vi "GA_DisplaySolution.vi"(5 "ClassifierClass.lvclass":refnum<class "ClassifierClass.lvclass">, 8 "Stop Notifier In":refnum<notifier>, 10 "Controls Refs":T1, 11 "Solution Notifier In":refnum<notifier>) -> ()   [LabVIEW 2016, in "GA.lvlib"]
uses:
  GA.lvlib
  GA_tSolution progress.ctl
  4. Accuracy Assessment for EEG Classification/_vlib/ClassifierClass.lvclass
  4. Accuracy Assessment for EEG Classification/_vlib/CU_DataTypes.ctl
  4. Accuracy Assessment for EEG Classification/Classifier.lvlib
panel:
  # "This VI is a part of BCI Design library, http://www.ru-bci.org \nCopyright © 2020, Sotnikov Peter, All rights reserved. License: GNU GPLv3"
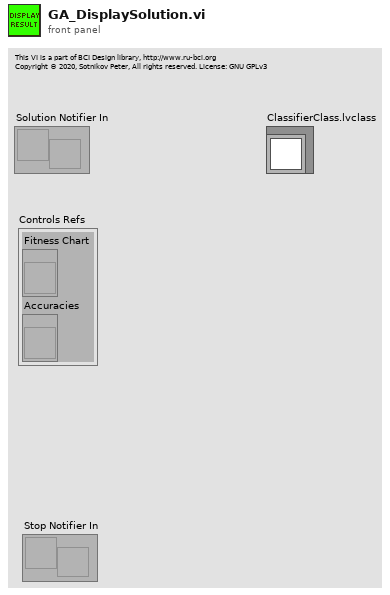
[diagram p1: front panel]
types:
  T1 = cluster{"Fitness Chart":refnum<vi>, "Accuracies":refnum<vi>}
  T2 = typedef "Classifier.lvlib/CU_DataTypes.ctl" = enum16{"Training Data", "Test Data", "Training Data (cross-check)", "Test Data (cross-check)"}
  T3 = typedef "GA.lvlib/GA_tSolution progress.ctl" = cluster{"Solution":i8[], "Fitness":dbl, "Mutation rate":dbl, "Generation":i32}
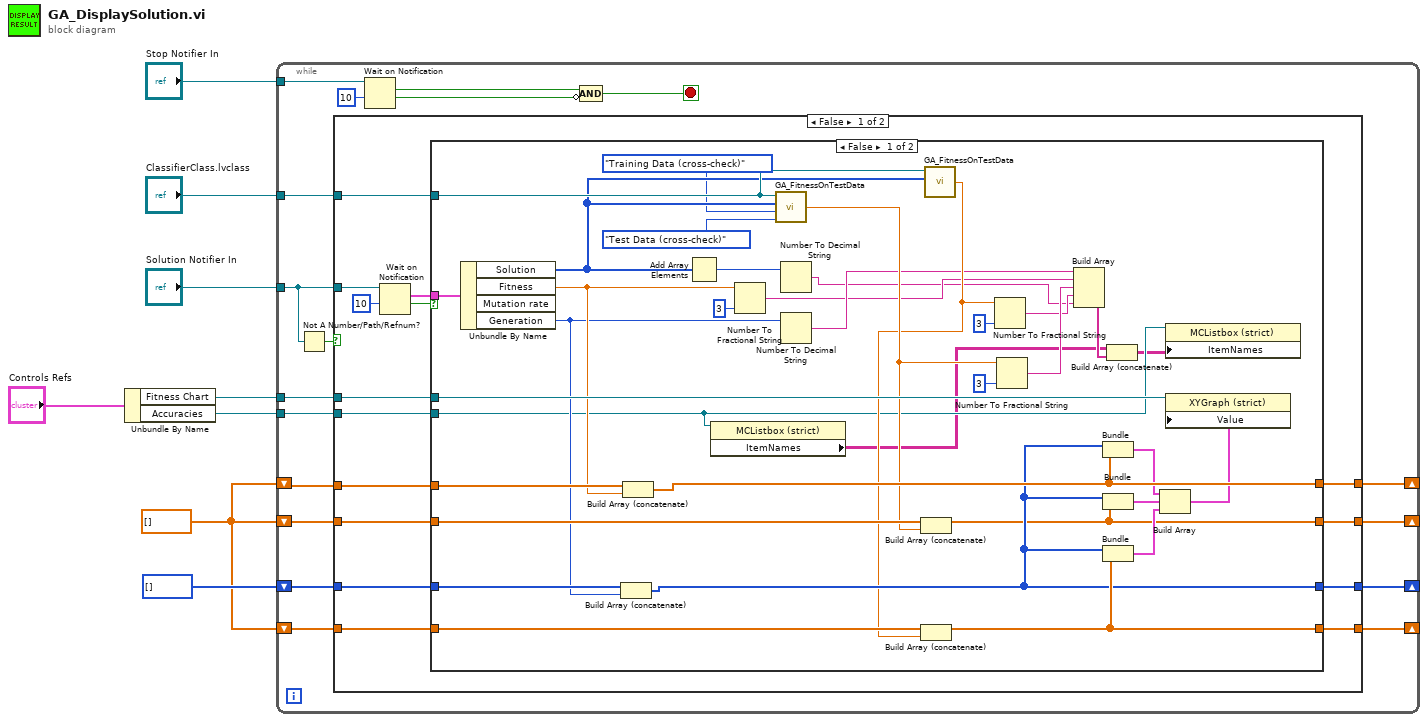
[diagram p0: block diagram]
diagram:
  w3 = dbl[] []
  n1 = Unbundle By Name("Controls Refs") -> ("Fitness Chart"=w6:refnum<vi>, "Accuracies"=w1:refnum<vi>)
  n2 = while {
    tunnel: "Solution Notifier In" -> [w25]
    tunnel: "Stop Notifier In" -> [w24]
    shift-right: [w18] -> _
    shift-left: w3 -> [w19]
    tunnel: w6 -> [w17]
    shift-right: [w14] -> _
    shift-left: i32[] [] -> [w16]
    shift-right: [w13] -> _
    shift-left: w3 -> [w15]
    tunnel: "ClassifierClass.lvclass" -> [w12]
    shift-right: [w10] -> _
    shift-left: w3 -> [w11]
    tunnel: w1 -> [w9]
    stop <- w20 stop-if-true
    n3 = Not A Number/Path/Refnum?(number/path/refnum=w25) -> (NaN/Path/Refnum?=w26:bool)
    n4 = case shown="False" w26 {
      tunnel: w25 -> [w41 _]
      tunnel: w19 -> [w37 w84]
      tunnel: [w36 w84] -> w18
      tunnel: w17 -> [w35 _]
      tunnel: w16 -> [w34 w83]
      tunnel: w15 -> [w33 w82]
      tunnel: [w32 w83] -> w14
      tunnel: [w31 w82] -> w13
      tunnel: w12 -> [w30 _]
      tunnel: w11 -> [w29 w81]
      tunnel: [w28 w81] -> w10
      tunnel: w9 -> [w27 _]
      frame False {
        n5 = Wait on Notification(notifier=w41, timeout in ms (-1)=10) -> (notification=w39:T3, timed out?=w40:bool)  [unwired: 2 in, 2 out]
        n6 = case shown="False" w40 {
          tunnel: w39 -> [w76 _]
          tunnel: w37 -> [w75 w80]
          tunnel: [w72 w80] -> w36
          tunnel: w35 -> [w60 _]
          tunnel: w34 -> [w74 w79]
          tunnel: w33 -> [w73 w78]
          tunnel: [w66 w79] -> w32
          tunnel: [w71 w78] -> w31
          tunnel: w30 -> [w62 _]
          tunnel: w29 -> [w67 w77]
          tunnel: [w64 w77] -> w28
          tunnel: w27 -> [w51 _]
          frame False {
            n7 = Unbundle By Name(w76) -> ("Solution"=w61:i8[], "Fitness"=w59:dbl, "Generation"=w54:i32)  [unwired: 1 out]
            n8 = Build Array (concatenate)(w74, w54) -> (w66:i32[])
            n9 = Build Array (concatenate)(w75, w59) -> (w72:dbl[])
            n10 = Add Array Elements(numeric array=w61) -> (sum=w57:i8)
            n11 = property class="MCListbox (strict)"(reference=w51) -> ("ItemNames"=w44:string[][])  [unwired: 1 in, 2 out]
            n12 = Number To Fractional String(number=w59, precision (6)=i16 3) -> (F-format string=w49:string)  [unwired: 2 in]
            n13 = call "GA_FitnessOnTestData.vi"("ClassifierClass.lvclass"=w62, "Phenotype"=w61, "TrainingData"=CU_DataTypes."Training Data (cross-check)", "TestData"=CU_DataTypes."Test Data (cross-check)") -> ("Fitness"=w53:dbl)  [unwired: 1 in]
            n14 = Number To Decimal String(number=w57) -> (decimal integer string=w46:string)  [unwired: 1 in]
            n15 = Number To Decimal String(number=w54) -> (decimal integer string=w50:string)  [unwired: 1 in]
            n16 = Build Array (concatenate)(w67, w53) -> (w64:dbl[])
            n17 = call "GA_FitnessOnTestData.vi"("ClassifierClass.lvclass"=w62, "Phenotype"=w61) -> ("Fitness"=w52:dbl)  [unwired: 3 in]
            n18 = Build Array (concatenate)(w73, w52) -> (w71:dbl[])
            n19 = Number To Fractional String(number=w52, precision (6)=i16 3) -> (F-format string=w47:string)  [unwired: 2 in]
            n20 = Number To Fractional String(number=w53, precision (6)=i16 3) -> (F-format string=w48:string)  [unwired: 2 in]
            n21 = Build Array(w50, w49, w48, w47, w46) -> (w45:string[])
            n22 = Bundle(w66, w72) -> (w70:cluster{i32[], dbl[]})  [unwired: 1 in]
            n23 = Bundle(w66, w64) -> (w65:cluster{i32[], dbl[]})  [unwired: 1 in]
            n24 = Bundle(w66, w71) -> (w68:cluster{i32[], dbl[]})  [unwired: 1 in]
            n25 = Build Array (concatenate)(w44, w45) -> (w43:string[][])
            n26 = Build Array(w70, w65, w68) -> (w69:cluster{i32[], dbl[]}[])
            n27 = property class="MCListbox (strict)"(reference=w51, "ItemNames"=w43) -> ()  [unwired: 1 in, 2 out]
            n28 = property class="XYGraph (strict)"(reference=w60, "Value"=w69) -> ()  [unwired: 1 in, 2 out]
          }
          frame True {
          }
        }
      }
      frame True {
      }
    }
    n29 = Wait on Notification(notifier=w24, timeout in ms (-1)=10) -> (notification=w22:bool, timed out?=w21:bool)  [unwired: 2 in, 2 out]
    n30 = Compound Arithmetic op=AND(w22, invert w21) -> (w20:bool)
  }
